vi "getTitle.vi"(8 "error in (no error)":errorcluster, 11 "Video in":refnum<class "Video.lvclass">) -> (0 "error out":errorcluster, 2 "title":string, 3 "Video out":refnum<class "Video.lvclass">)   [LabVIEW 2017, in "Video.lvclass"]
uses:
  Video.lvclass
  Video.lvclass/Video.ctl
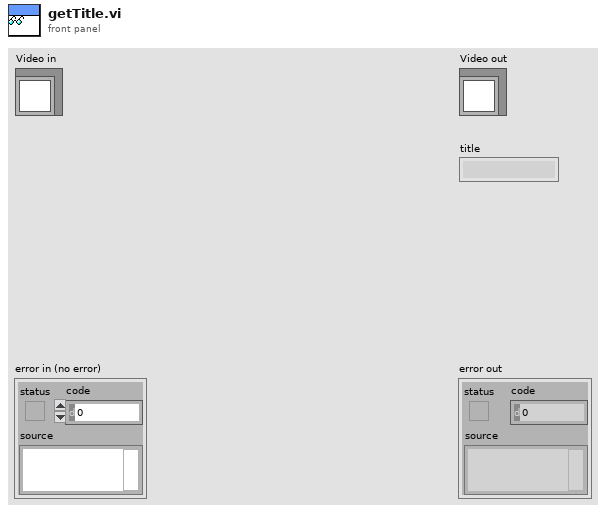
[diagram p1: front panel]
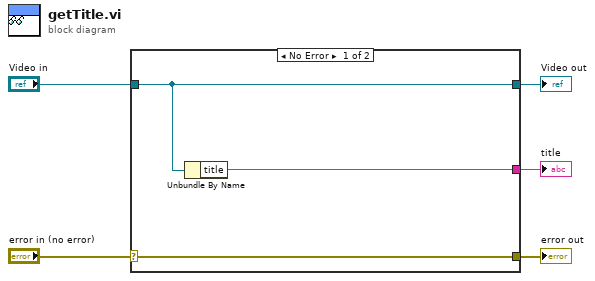
[diagram p0: block diagram]
diagram:
  n1 = case shown="No Error" "error in (no error)" {
    selector: "error in (no error)" -> [w8 w9]
    tunnel: [w8 w9] -> w4
    tunnel: [w7 w10] -> w2
    tunnel: "Video in" -> [w7 w10]
    tunnel: [w6 _] -> w1
    frame No Error {
      n2 = Unbundle By Name(w7) -> ("title"=w6:string)
    }
    frame Error {
    }
  }
  "error out" <- w4
  "Video out" <- w2
  "title" <- w1
